vi "Thermocouple.vi"(7 "Thermocouple channels":string, 8 "Start measure = True":bool) -> (2 "Reference temperature":dbl[](array[numeric]))   [LabVIEW 2021]
panel:
  in  "Numeric":i32=1
  out "error out":errorcluster
  in  "VISA":refnum<visa-resource-name>="USB0::2391::1287::MY44008368::0::INSTR"
  in  "error in (no error)":errorcluster
  out "Thermocouple":dbl[](array[numeric])
  in  "Thermocouple Type":T1(ring)=enum."K-Type"
  in  "Measurements per channel":i32=3 min=1 max=1000
  out "Unedited measurement data":dbl[](array[numeric])
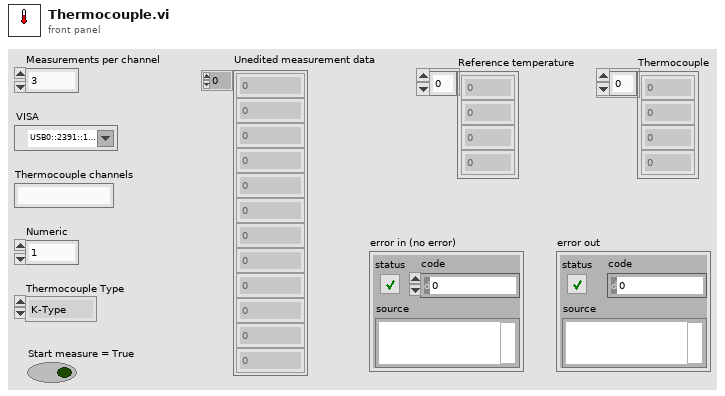
[diagram p1: front panel]
types:
  T1 = enum16{"B-Type", "E-Type", "J-Type", "K-Type", "N-Type", "R-Type", "S-Type", "T-Type"}
  T2 = enum16{"Bus", "Immediate", "External", "Alarm 1", "Alarm 2", "Alarm 3", "Alarm 4", "Timer"}
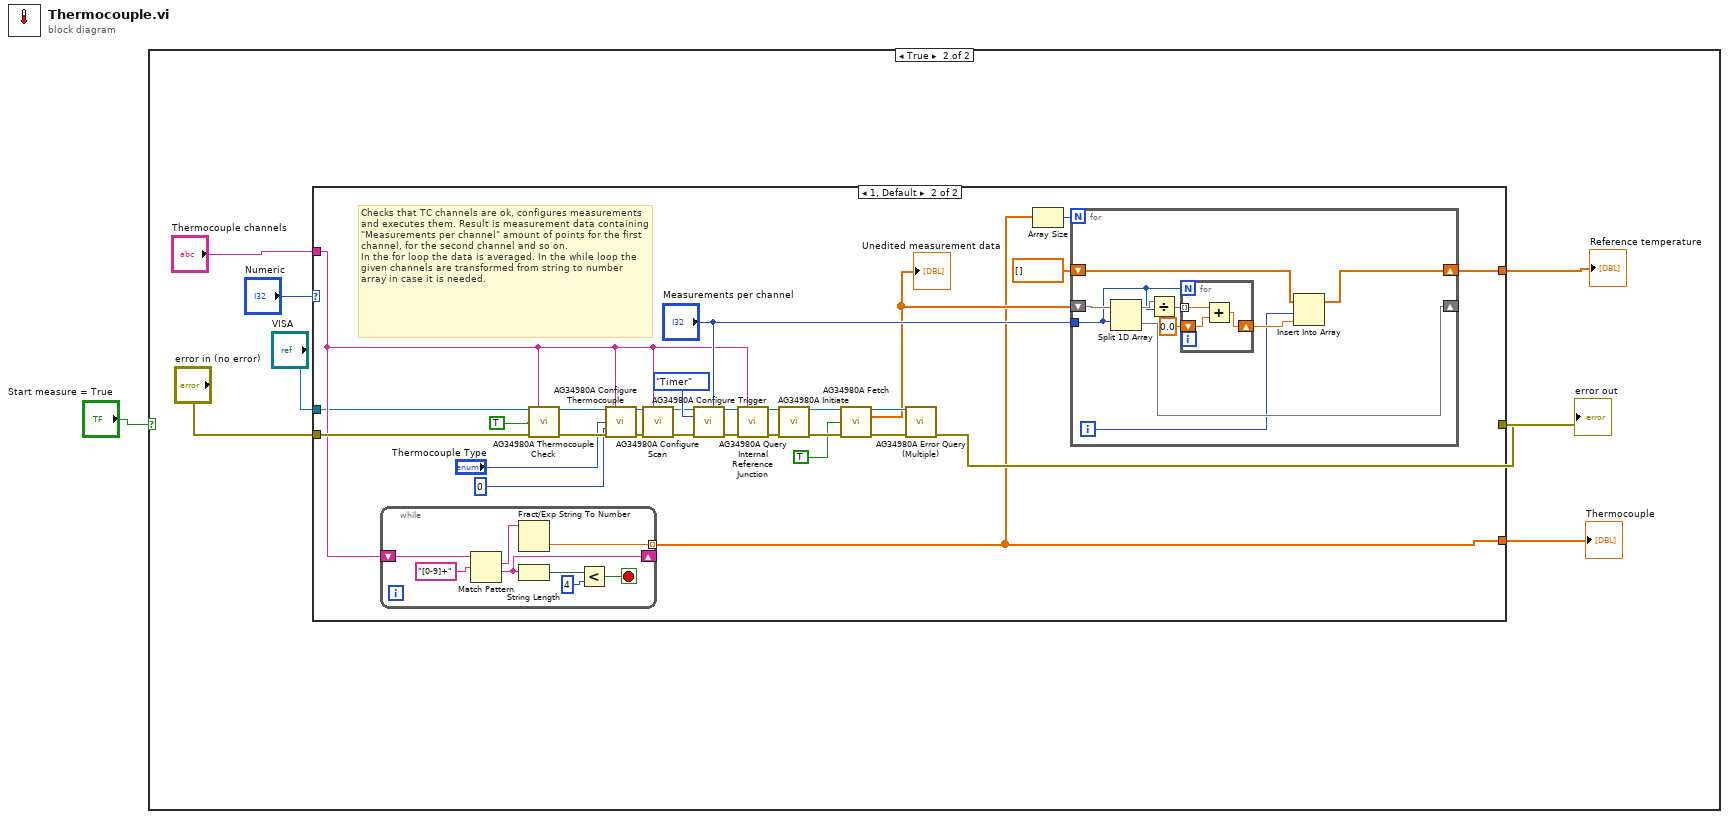
[diagram p0: block diagram]
diagram:
  n1 = case shown="True" "Start measure = True" {
    frame False {
    }
    frame True {
      n2 = case shown="1, Default" "Numeric" {
        tunnel: "Thermocouple channels" -> [_ w14]
        tunnel: "error in (no error)" -> [w9 w20]
        tunnel: [w9 w19] -> w6
        tunnel: "VISA" -> [_ w12]
        tunnel: [_ w11] -> w3
        tunnel: [_ w10] -> w2
        frame 0 {
        }
        frame 1, Default {
          # "Checks that TC channels are ok, configures measurements and executes them. Result is measurement data containing \"Measurements per channel\" amount of points for the first channel, for the second channel and so on.\nIn the for loop the data is averaged. In the while loop the given channels are transformed from string to number array in case it is needed."
          n3 = while {
            shift-right: [w39] -> _
            shift-left: w14 -> [w42]
            tunnel: [w41] -> w11 mode=indexing
            stop <- w40 stop-if-true
            n4 = Match Pattern(string=w42, regular expression="[0-9]+" ("Thermocouple channels")) -> (match substring=w46:string, after substring=w39:string)  [unwired: 1 in, 2 out]
            n5 = Fract/Exp String To Number(string=w46) -> (number=w41:dbl)  [unwired: 3 in, 1 out]
            n6 = String Length(string=w39) -> (length=w44:i32)
            n7 = Less?(x=w44, y=4) -> (x < y?=w40:bool)
          }
          n8 = call "AG34980A Thermocouple Check.vi"("VISA resource name"=w12, "Channel List(empty)"=w14, "Enable (F:Disable)"=TRUE, "error in (no error)"=w20) -> ("VISA resource name out"=w36:refnum<visa-resource-name>, "error out"=w37:errorcluster)  [unwired: 10 in]
          n9 = call "AG34980A Configure Thermocouple.vi"("VISA resource name"=w36, "Channel List(empty)"=w14, "Thermocouple Type (2:J-Type)"="Thermocouple Type", "Reference Junction Type (2:Fixed)"=0, "error in (no error)"=w37) -> ("VISA resource name out"=w33:refnum<visa-resource-name>, "error out"=w32:errorcluster)  [unwired: 9 in]
          n10 = call "AG34980A Configure Scan.vi"("VISA resource name"=w33, "Scan List(empty)"=w14, "error in (no error)"=w32) -> ("VISA resource name out"=w16:refnum<visa-resource-name>, "error out"=w31:errorcluster)  [unwired: 11 in]
          n11 = call "AG34980A Configure Trigger.vi"("VISA resource name"=w16, "Sample Count (1)"="Measurements per channel", "Trigger Source (1:Immediate)"=T2."Timer", "error in (no error)"=w31) -> ("VISA resource name out"=w34:refnum<visa-resource-name>, "error out"=w35:errorcluster)  [unwired: 10 in]
          n12 = call "AG34980A Query Internal Reference Junction.vi"("VISA resource name"=w34, "Channel List"=w14, "error in (no error)"=w35) -> ("VISA resource name out"=w25:refnum<visa-resource-name>, "error out"=w24:errorcluster)  [unwired: 10 in, 1 out]
          n13 = call "AG34980A Initiate.vi"("VISA resource name"=w25, "error in (no error)"=w24) -> ("VISA resource name out"=w21:refnum<visa-resource-name>, "error out"=w27:errorcluster)  [unwired: 12 in]
          n14 = call "AG34980A Fetch.vi"("VISA resource name"=w21, "Numbers Only (T:On)"=TRUE, "error in (no error)"=w27) -> ("VISA resource name out"=w23:refnum<visa-resource-name>, "Output Data (Numbers Only)"=w13:dbl[], "error out"=w22:errorcluster)  [unwired: 9 in, 1 out]
          "Unedited measurement data" <- w13
          n15 = call "AG34980A Error Query (Multiple).vi"("VISA resource name"=w23, "error in (no error)"=w22) -> ("error out"=w19:errorcluster)  [unwired: 10 in, 3 out]
          n16 = Array Size(array=w11) -> (size(s)=w15:i32)
          n17 = for {
            N: w15 -> [_]
            shift-right: [w55] -> _
            shift-left: w13 -> [w56]
            shift-right: [w48] -> w10
            shift-left: dbl[] [] ("Reference temperature") -> [w49]
            tunnel: "Measurements per channel" -> [w47]
            i -> [w50]
            n18 = Split 1D Array(array=w56, index=w47) -> (first subarray=w52:dbl[], second subarray=w55:dbl[])
            n19 = Divide(x=w52, y=w47) -> (x/y=w53:dbl[])
            n20 = for {
              N: w47 -> [_]
              shift-right: [w57] -> w51
              shift-left: 0.0 ("index") -> [w59]
              tunnel: w53 -> [w58] mode=indexing
              n21 = Add(x=w58, y=w59) -> (x+y=w57:dbl)
            }
            n22 = Insert Into Array(array=w49, index=w50, new element=w51) -> (w48:dbl[])
          }
        }
      }
      "Reference temperature" <- w2
      "Thermocouple" <- w3
      "error out" <- w6
    }
  }
